vi "PicoLogStart_2.vi"(0 "Ch nr":bool[](array[boolean]), 1 "Single ended\n(0- single)\n(1 - difer)":i32[](array[numeric]) min=0 max=1 step=1, 2 "Voltage range":i32[](array[numeric]) min=0 max=6 step=1, 3 "sampleInterval_ms":i32=1000, 5 "conversionTime":i16(ring) items=["60 ms", "100 ms", "180 ms", "340 ms", "660 ms"], 6 "Mains Frequency":i16(ring) items=["50 Hz", "60 Hz"]) -> (4 "noOfChannels":i16=2, 7 "handle":i16, 8 "STOP":bool)   [LabVIEW 2014]
uses:
  Instance           1 22Saved   HRDL_streaming .vi
  Instance         138 22Saved   HRDL_streaming .vi
  picohrdl.dll
panel:
  out "Unit Info":T1
  # "1       2       3      4       5        6       7       8       9      10     11      12     13    14       15     16"
  # "0 -+2500mV\n1 -+1250mV\n2 -+625mV\n3 -+313mV\n4 -+156mV\n5 -+78mv\n6 -+39mV"
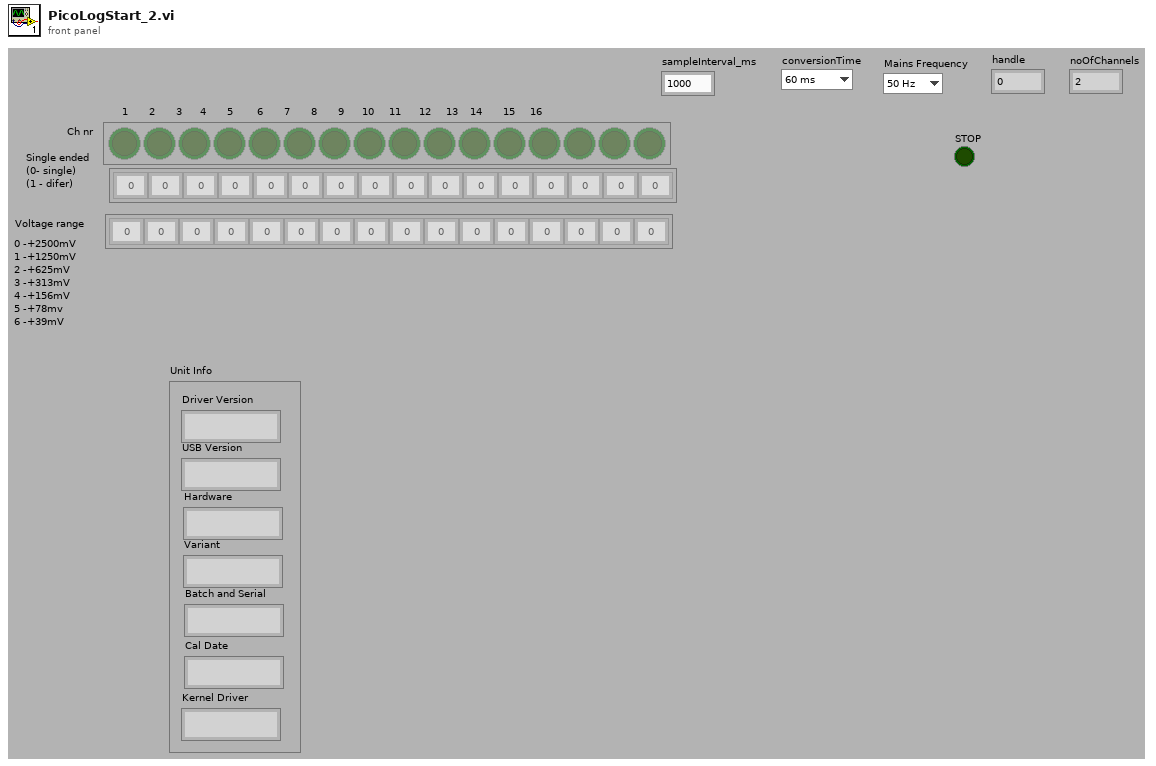
[diagram p1: front panel]
types:
  T1 = cluster{"Driver Version":string, "USB Version":string, "Hardware":string, "Variant":string, "Batch and Serial":string, "Cal Date":string, "Kernel Driver":string}
  T2 = cluster{"[0]":string, "[1]":string, "[2]":string, "[3]":string, "[4]":string, "[5]":string, "[6]":string}
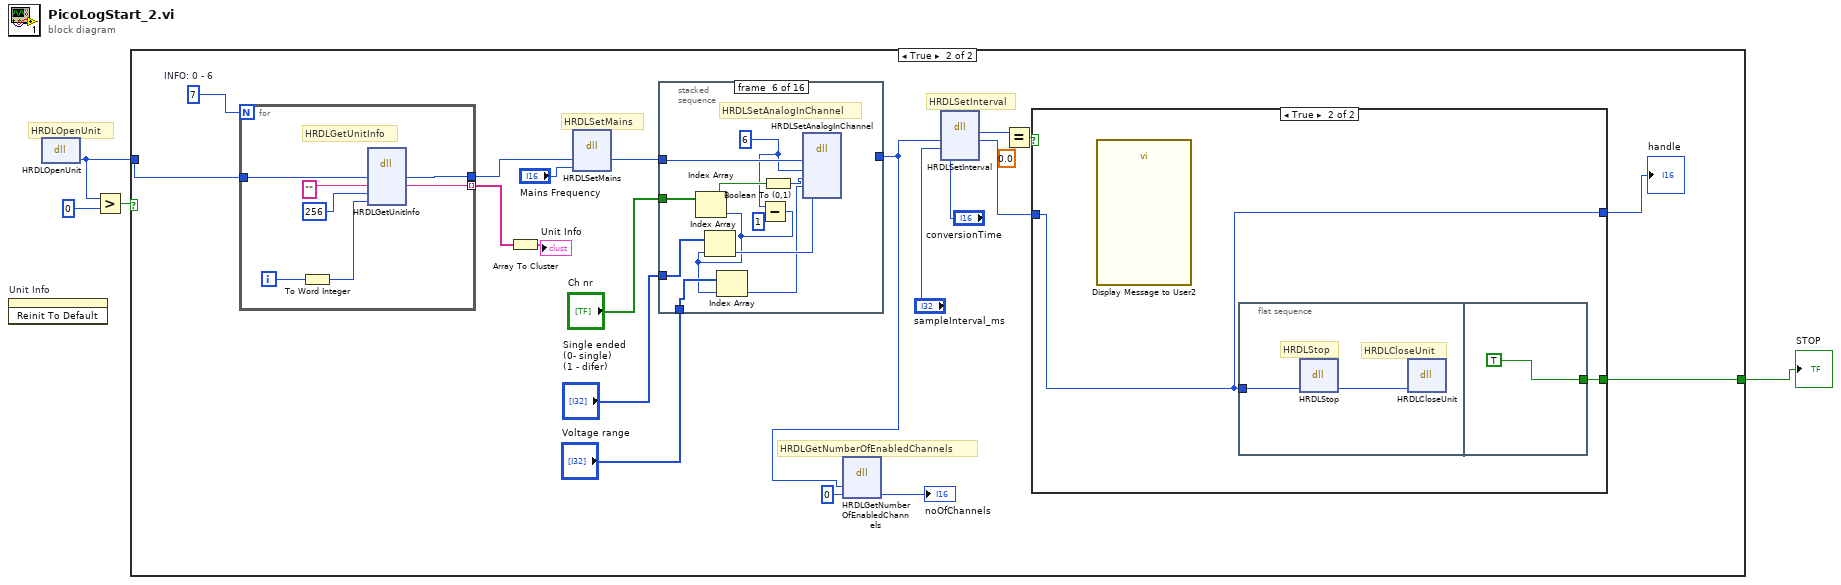
[diagram p0: block diagram]
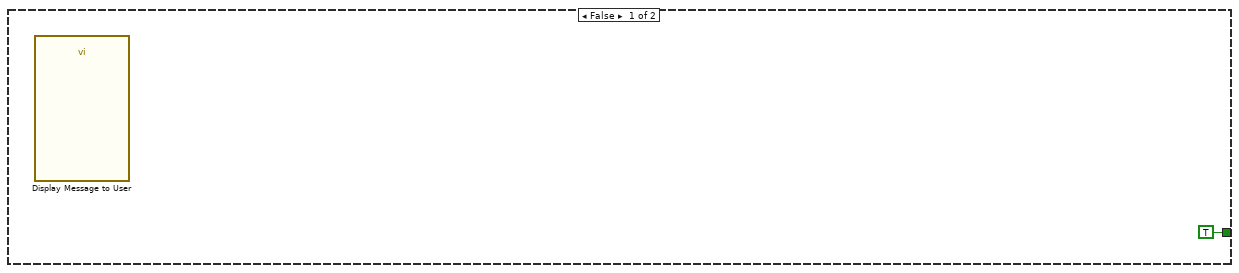
[diagram p2: hidden frame]
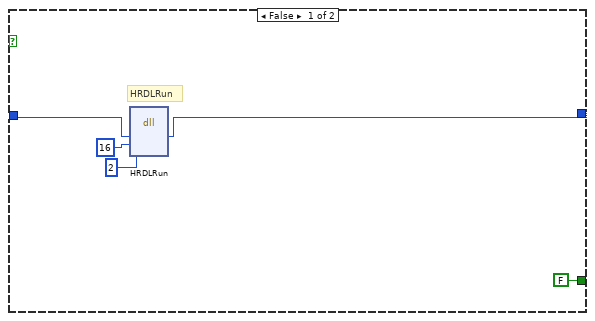
[diagram p3: hidden frame]
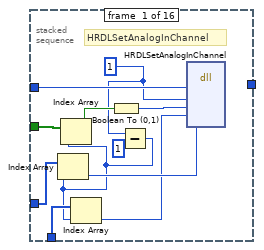
[diagram p4: hidden frame]
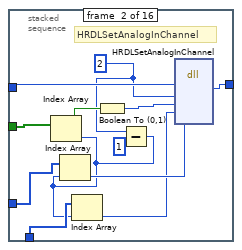
[diagram p5: hidden frame]
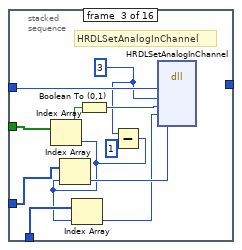
[diagram p6: hidden frame]
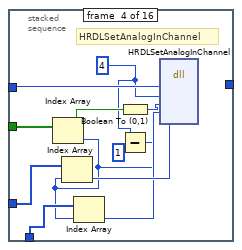
[diagram p7: hidden frame]
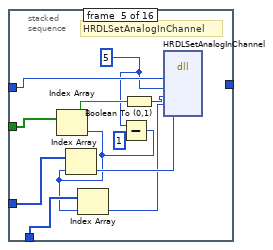
[diagram p8: hidden frame]
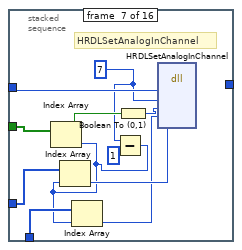
[diagram p9: hidden frame]
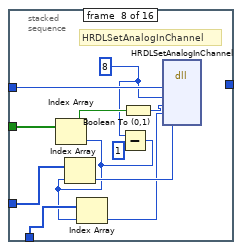
[diagram p10: hidden frame]
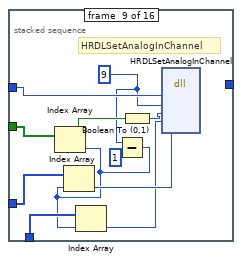
[diagram p11: hidden frame]
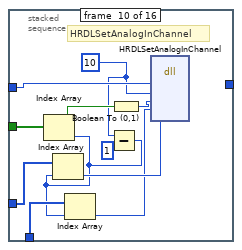
[diagram p12: hidden frame]
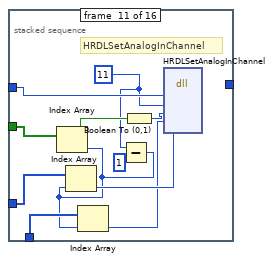
[diagram p13: hidden frame]
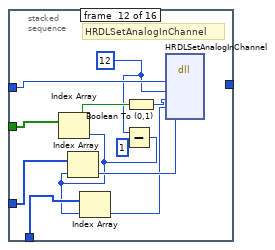
[diagram p14: hidden frame]
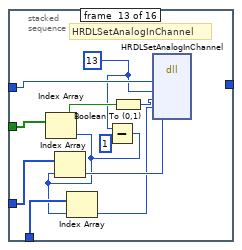
[diagram p15: hidden frame]
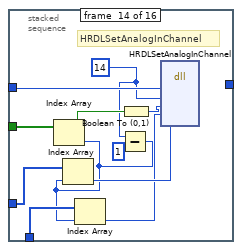
[diagram p16: hidden frame]
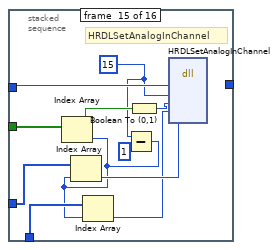
[diagram p17: hidden frame]
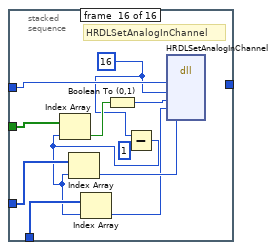
[diagram p18: hidden frame]
diagram:
  # "HRDLOpenUnit"
  n1 = invoke on="Unit Info" class="Clust (strict)" method="Reinit To Default"() -> ()  [unwired: 3 in, 3 out]
  n2 = dll-call lib="picohrdl.dll" fn="HRDLOpenUnit"() -> ("handle"=w2:i16)  [unwired: 3 in, 2 out]
  n3 = Greater?(x=w2, y=i16 0) -> (0:w4:bool)
  n4 = case shown="True" w4 {
    tunnel: w2 -> [_ w17]
    tunnel: [TRUE ("stop") w8] -> w1
    frame False {
      n5 = call "Display Message to User"() -> ()  [unwired: 10 in, 2 out]
    }
    frame True {
      w19 = 7  # INFO: 0 - 6
      # "HRDLGetNumberOfEnabledChannels"
      # "HRDLSetInterval"
      # "HRDLSetMains"
      n6 = for {
        N: w19 -> [_]
        tunnel: w17 -> [w33]
        tunnel: [w30] -> w16 mode=indexing
        tunnel: [w28] -> w18
        i -> [w29]
        # "HRDLGetUnitInfo"
        n7 = To Word Integer(number=w29) -> (16bit integer=w27:i16)
        n8 = dll-call lib="picohrdl.dll" fn="HRDLGetUnitInfo"("handle"=w33, "unitInfo"="", "stringLength"=i16 256, "info"=w27) -> ("handle"=w28:i16, "unitInfo"=w30:string)  [unwired: 6 in, 2 out]
      }
      n9 = Array To Cluster(array=w16) -> (cluster=→"Unit Info":T2)
      n10 = dll-call lib="PicoHRDL.dll" fn="HRDLSetMains"("handle"=w18, "sixtyHertz"="Mains Frequency") -> ("handle"=w7:i16)  [unwired: 5 in, 2 out]
      n11 = stacked-sequence {
        tunnel: w7 -> [w54 w62 w73 w81 w95 w106 w117 w128 w139 w150 w161 w172 w183 w194 w205 w216]
        tunnel: "Ch nr" -> [w52 w61 w72 w84 w94 w105 w116 w127 w138 w149 w160 w171 w182 w193 w204 w215]
        tunnel: "Single ended\n(0- single)\n(1 - difer)" -> [w50 w60 w71 w82 w93 w104 w115 w126 w137 w148 w159 w170 w181 w192 w203 w214]
        tunnel: "Voltage range" -> [w48 w59 w70 w83 w92 w103 w114 w125 w136 w147 w158 w169 w180 w191 w202 w213]
        tunnel: [_ w55 _ _ _ _ _ _ _ _ _ _ _ _ _ _] -> w6
        frame #0 {
          w46 = i16 1 ("channel")
          # "HRDLSetAnalogInChannel"
          n12 = Subtract(x=w46, y=i16 1) -> (x-y=w45:i16)
          n13 = Index Array(array=w50, index=w45) -> (element=w49:i32)
          n14 = Index Array(array=w52, index=w45) -> (element=w51:bool)
          n15 = Index Array(array=w48, index=w45) -> (element=w47:i32)
          n16 = Boolean To (0,1)(Boolean=w51) -> (0, 1=w53:i16)
          n17 = dll-call lib="PicoHRDL.dll" fn="HRDLSetAnalogInChannel"("handle"=w54, "channel"=w46, "enabled"=w53, "range"=w47, "singleEnded"=w49) -> ()  [unwired: 9 in, 2 out]
        }
        frame #1 {
          w57 = i16 2 ("channel")
          # "HRDLSetAnalogInChannel"
          n18 = Subtract(x=w57, y=i16 1) -> (x-y=w56:i16)
          n19 = Index Array(array=w61, index=w56) -> (element=w65:bool)
          n20 = Index Array(array=w60, index=w56) -> (element=w64:i32)
          n21 = Index Array(array=w59, index=w56) -> (element=w63:i32)
          n22 = Boolean To (0,1)(Boolean=w65) -> (0, 1=w66:i16)
          n23 = dll-call lib="PicoHRDL.dll" fn="HRDLSetAnalogInChannel"("handle"=w62, "channel"=w57, "enabled"=w66, "range"=w63, "singleEnded"=w64) -> ("handle"=w55:i16)  [unwired: 8 in, 2 out]
        }
        frame #2 {
          w68 = i16 3 ("channel")
          # "HRDLSetAnalogInChannel"
          n24 = Subtract(x=w68, y=i16 1) -> (x-y=w67:i16)
          n25 = Index Array(array=w72, index=w67) -> (element=w76:bool)
          n26 = Index Array(array=w71, index=w67) -> (element=w75:i32)
          n27 = Index Array(array=w70, index=w67) -> (element=w74:i32)
          n28 = Boolean To (0,1)(Boolean=w76) -> (0, 1=w77:i16)
          n29 = dll-call lib="PicoHRDL.dll" fn="HRDLSetAnalogInChannel"("handle"=w73, "channel"=w68, "enabled"=w77, "range"=w74, "singleEnded"=w75) -> ()  [unwired: 9 in, 2 out]
        }
        frame #3 {
          w79 = i16 4 ("channel")
          # "HRDLSetAnalogInChannel"
          n30 = Subtract(x=w79, y=i16 1) -> (x-y=w78:i16)
          n31 = Index Array(array=w84, index=w78) -> (element=w87:bool)
          n32 = Index Array(array=w82, index=w78) -> (element=w86:i32)
          n33 = Index Array(array=w83, index=w78) -> (element=w85:i32)
          n34 = Boolean To (0,1)(Boolean=w87) -> (0, 1=w88:i16)
          n35 = dll-call lib="PicoHRDL.dll" fn="HRDLSetAnalogInChannel"("handle"=w81, "channel"=w79, "enabled"=w88, "range"=w85, "singleEnded"=w86) -> ()  [unwired: 9 in, 2 out]
        }
        frame #4 {
          w90 = i16 5 ("channel")
          # "HRDLSetAnalogInChannel"
          n36 = Subtract(x=w90, y=i16 1) -> (x-y=w89:i16)
          n37 = Index Array(array=w94, index=w89) -> (element=w98:bool)
          n38 = Index Array(array=w93, index=w89) -> (element=w97:i32)
          n39 = Index Array(array=w92, index=w89) -> (element=w96:i32)
          n40 = Boolean To (0,1)(Boolean=w98) -> (0, 1=w99:i16)
          n41 = dll-call lib="PicoHRDL.dll" fn="HRDLSetAnalogInChannel"("handle"=w95, "channel"=w90, "enabled"=w99, "range"=w96, "singleEnded"=w97) -> ()  [unwired: 9 in, 2 out]
        }
        frame #5 {
          w101 = i16 6 ("channel")
          # "HRDLSetAnalogInChannel"
          n42 = Subtract(x=w101, y=i16 1) -> (x-y=w100:i16)
          n43 = Index Array(array=w105, index=w100) -> (element=w109:bool)
          n44 = Index Array(array=w104, index=w100) -> (element=w108:i32)
          n45 = Index Array(array=w103, index=w100) -> (element=w107:i32)
          n46 = Boolean To (0,1)(Boolean=w109) -> (0, 1=w110:i16)
          n47 = dll-call lib="PicoHRDL.dll" fn="HRDLSetAnalogInChannel"("handle"=w106, "channel"=w101, "enabled"=w110, "range"=w107, "singleEnded"=w108) -> ()  [unwired: 9 in, 2 out]
        }
        frame #6 {
          w112 = i16 7 ("channel")
          # "HRDLSetAnalogInChannel"
          n48 = Subtract(x=w112, y=i16 1) -> (x-y=w111:i16)
          n49 = Index Array(array=w116, index=w111) -> (element=w120:bool)
          n50 = Index Array(array=w115, index=w111) -> (element=w119:i32)
          n51 = Index Array(array=w114, index=w111) -> (element=w118:i32)
          n52 = Boolean To (0,1)(Boolean=w120) -> (0, 1=w121:i16)
          n53 = dll-call lib="PicoHRDL.dll" fn="HRDLSetAnalogInChannel"("handle"=w117, "channel"=w112, "enabled"=w121, "range"=w118, "singleEnded"=w119) -> ()  [unwired: 9 in, 2 out]
        }
        frame #7 {
          w123 = i16 8 ("channel")
          # "HRDLSetAnalogInChannel"
          n54 = Subtract(x=w123, y=i16 1) -> (x-y=w122:i16)
          n55 = Index Array(array=w127, index=w122) -> (element=w131:bool)
          n56 = Index Array(array=w126, index=w122) -> (element=w130:i32)
          n57 = Index Array(array=w125, index=w122) -> (element=w129:i32)
          n58 = Boolean To (0,1)(Boolean=w131) -> (0, 1=w132:i16)
          n59 = dll-call lib="PicoHRDL.dll" fn="HRDLSetAnalogInChannel"("handle"=w128, "channel"=w123, "enabled"=w132, "range"=w129, "singleEnded"=w130) -> ()  [unwired: 9 in, 2 out]
        }
        frame #8 {
          w134 = i16 9 ("channel")
          # "HRDLSetAnalogInChannel"
          n60 = Subtract(x=w134, y=i16 1) -> (x-y=w133:i16)
          n61 = Index Array(array=w138, index=w133) -> (element=w142:bool)
          n62 = Index Array(array=w137, index=w133) -> (element=w141:i32)
          n63 = Index Array(array=w136, index=w133) -> (element=w140:i32)
          n64 = Boolean To (0,1)(Boolean=w142) -> (0, 1=w143:i16)
          n65 = dll-call lib="PicoHRDL.dll" fn="HRDLSetAnalogInChannel"("handle"=w139, "channel"=w134, "enabled"=w143, "range"=w140, "singleEnded"=w141) -> ()  [unwired: 9 in, 2 out]
        }
        frame #9 {
          w145 = i16 10 ("channel")
          # "HRDLSetAnalogInChannel"
          n66 = Subtract(x=w145, y=i16 1) -> (x-y=w144:i16)
          n67 = Index Array(array=w149, index=w144) -> (element=w153:bool)
          n68 = Index Array(array=w148, index=w144) -> (element=w152:i32)
          n69 = Index Array(array=w147, index=w144) -> (element=w151:i32)
          n70 = Boolean To (0,1)(Boolean=w153) -> (0, 1=w154:i16)
          n71 = dll-call lib="PicoHRDL.dll" fn="HRDLSetAnalogInChannel"("handle"=w150, "channel"=w145, "enabled"=w154, "range"=w151, "singleEnded"=w152) -> ()  [unwired: 9 in, 2 out]
        }
        frame #10 {
          w156 = i16 11 ("channel")
          # "HRDLSetAnalogInChannel"
          n72 = Subtract(x=w156, y=i16 1) -> (x-y=w155:i16)
          n73 = Index Array(array=w160, index=w155) -> (element=w164:bool)
          n74 = Index Array(array=w159, index=w155) -> (element=w163:i32)
          n75 = Index Array(array=w158, index=w155) -> (element=w162:i32)
          n76 = Boolean To (0,1)(Boolean=w164) -> (0, 1=w165:i16)
          n77 = dll-call lib="PicoHRDL.dll" fn="HRDLSetAnalogInChannel"("handle"=w161, "channel"=w156, "enabled"=w165, "range"=w162, "singleEnded"=w163) -> ()  [unwired: 9 in, 2 out]
        }
        frame #11 {
          w167 = i16 12 ("channel")
          # "HRDLSetAnalogInChannel"
          n78 = Subtract(x=w167, y=i16 1) -> (x-y=w166:i16)
          n79 = Index Array(array=w171, index=w166) -> (element=w175:bool)
          n80 = Index Array(array=w170, index=w166) -> (element=w174:i32)
          n81 = Index Array(array=w169, index=w166) -> (element=w173:i32)
          n82 = Boolean To (0,1)(Boolean=w175) -> (0, 1=w176:i16)
          n83 = dll-call lib="PicoHRDL.dll" fn="HRDLSetAnalogInChannel"("handle"=w172, "channel"=w167, "enabled"=w176, "range"=w173, "singleEnded"=w174) -> ()  [unwired: 9 in, 2 out]
        }
        frame #12 {
          w178 = i16 13 ("channel")
          # "HRDLSetAnalogInChannel"
          n84 = Subtract(x=w178, y=i16 1) -> (x-y=w177:i16)
          n85 = Index Array(array=w182, index=w177) -> (element=w186:bool)
          n86 = Index Array(array=w181, index=w177) -> (element=w185:i32)
          n87 = Index Array(array=w180, index=w177) -> (element=w184:i32)
          n88 = Boolean To (0,1)(Boolean=w186) -> (0, 1=w187:i16)
          n89 = dll-call lib="PicoHRDL.dll" fn="HRDLSetAnalogInChannel"("handle"=w183, "channel"=w178, "enabled"=w187, "range"=w184, "singleEnded"=w185) -> ()  [unwired: 9 in, 2 out]
        }
        frame #13 {
          w189 = i16 14 ("channel")
          # "HRDLSetAnalogInChannel"
          n90 = Subtract(x=w189, y=i16 1) -> (x-y=w188:i16)
          n91 = Index Array(array=w193, index=w188) -> (element=w197:bool)
          n92 = Index Array(array=w192, index=w188) -> (element=w196:i32)
          n93 = Index Array(array=w191, index=w188) -> (element=w195:i32)
          n94 = Boolean To (0,1)(Boolean=w197) -> (0, 1=w198:i16)
          n95 = dll-call lib="PicoHRDL.dll" fn="HRDLSetAnalogInChannel"("handle"=w194, "channel"=w189, "enabled"=w198, "range"=w195, "singleEnded"=w196) -> ()  [unwired: 9 in, 2 out]
        }
        frame #14 {
          w200 = i16 15 ("channel")
          # "HRDLSetAnalogInChannel"
          n96 = Subtract(x=w200, y=i16 1) -> (x-y=w199:i16)
          n97 = Index Array(array=w204, index=w199) -> (element=w208:bool)
          n98 = Index Array(array=w203, index=w199) -> (element=w207:i32)
          n99 = Index Array(array=w202, index=w199) -> (element=w206:i32)
          n100 = Boolean To (0,1)(Boolean=w208) -> (0, 1=w209:i16)
          n101 = dll-call lib="PicoHRDL.dll" fn="HRDLSetAnalogInChannel"("handle"=w205, "channel"=w200, "enabled"=w209, "range"=w206, "singleEnded"=w207) -> ()  [unwired: 9 in, 2 out]
        }
        frame #15 {
          w211 = i16 16 ("channel")
          # "HRDLSetAnalogInChannel"
          n102 = Subtract(x=w211, y=i16 1) -> (x-y=w210:i16)
          n103 = Index Array(array=w215, index=w210) -> (element=w219:bool)
          n104 = Index Array(array=w214, index=w210) -> (element=w218:i32)
          n105 = Index Array(array=w213, index=w210) -> (element=w217:i32)
          n106 = Boolean To (0,1)(Boolean=w219) -> (0, 1=w220:i16)
          n107 = dll-call lib="PicoHRDL.dll" fn="HRDLSetAnalogInChannel"("handle"=w216, "channel"=w211, "enabled"=w220, "range"=w217, "singleEnded"=w218) -> ()  [unwired: 9 in, 2 out]
        }
      }
      n108 = dll-call lib="PicoHRDL.dll" fn="HRDLGetNumberOfEnabledChannels"("handle"=w6, "nEnabledChannels"=i16 0) -> ("nEnabledChannels"=→"noOfChannels":i16)  [unwired: 5 in, 2 out]
      n109 = dll-call lib="PicoHRDL.dll" fn="HRDLSetInterval"("handle"=w6, "sampleInterval_ms"="sampleInterval_ms", "conversionTime"="conversionTime") -> ("return type"=w23:i16, "handle"=w22:i16)  [unwired: 5 in, 2 out]
      n110 = Equal?(x=w23, y=0.0) -> (x = y?=w21:bool)
      n111 = case shown="True" w21 {
        tunnel: [w35 w40] -> w14
        tunnel: w22 -> [w36 w40]
        tunnel: [FALSE ("stop") w39] -> w8
        frame False {
          # "HRDLRun"
          n112 = dll-call lib="PicoHRDL.dll" fn="HRDLRun"("handle"=w36, "nValues"=16, "method"=i16 2) -> ("handle"=w35:i16)  [unwired: 6 in, 2 out]
        }
        frame True {
          n113 = call "Display Message to User2"() -> ()  [unwired: 10 in, 2 out]
          n114 = flat-sequence {
            tunnel: w40 -> [w41]
            tunnel: [TRUE ("stop")] -> w39
            frame #0 {
              # "HRDLStop"
              # "HRDLCloseUnit"
              n115 = dll-call lib="picohrdl.dll" fn="HRDLStop"("handle"=w41) -> ("handle"=w42:i16)  [unwired: 4 in, 2 out]
              n116 = dll-call lib="PicoHRDL.dll" fn="HRDLCloseUnit"("handle"=w42) -> ()  [unwired: 5 in, 2 out]
            }
            frame #1 {
            }
          }
        }
      }
      "handle" <- w14
    }
  }
  "STOP" <- w1
